vi "orderbook.test.Reduce.Size.1st.of.2.vi"(8 "error in":errorcluster) -> (0 "error out":errorcluster, 3 "Passed":bool)   [LabVIEW 2022 SP3]
uses:
  fpga/common/orderbook.command.type.ctl
  fpga/common/orderbook.command.ctl
  fpga/app/orderbook.result.type.ctl
  fpga/app/orderbook.entry.ctl
panel:
  out "Counters":T1
  out "OrderBook.Entries":T2[](array[typedef]) {"Side (U8)" format="%.0x"}
  in  "OrderBook.Command[]\nto Send":T4[](array[typedef])=[{"OrderBook Command.Type"=enum."AddOrder", "Side (U8)"=66, "Order Id (U64)"=336, "Quantity (U32)"=130, "Symbol (U64)"=29033, "Price (U64)"=9525, "Executed Quantity (U32)"=0, "Canceled Quantity (U32)"=0, "Remaining Quantity (U32)"=0, "Seconds (U64)"=0, "Nanoseconds (U64)"=0}, {"OrderBook Command.Type"=enum."AddOrder", "Side (U8)"=66, "Order Id (U64)"=337, "Quantity (U32)"=225, "Symbol (U64)"=29033, "Price (U64)"=9115, "Executed Quantity (U32)"=0, "Canceled Quantity (U32)"=0, "Remaining Quantity (U32)"=0, "Seconds (U64)"=0, "Nanoseconds (U64)"=0}, {"OrderBook Command.Type"=enum."ReduceSize", "Side (U8)"=66, "Order Id (U64)"=337, "Quantity (U32)"=0, "Symbol (U64)"=0, "Price (U64)"=0, "Executed Quantity (U32)"=0, "Canceled Quantity (U32)"=25, "Remaining Quantity (U32)"=0, "Seconds (U64)"=0, "Nanoseconds (U64)"=0}, {"OrderBook Command.Type"=enum."Get.All.Orders", "Side (U8)"=0, "Order Id (U64)"=0, "Quantity (U32)"=0, "Symbol (U64)"=0, "Price (U64)"=0, "Executed Quantity (U32)"=0, "Canceled Quantity (U32)"=0, "Remaining Quantity (U32)"=0, "Seconds (U64)"=0, "Nanoseconds (U64)"=0}] {"Side (U8)" format="%.0x"; "Order Id (U64)" format="%.0x"; "Symbol (U64)" format="%.0x"}
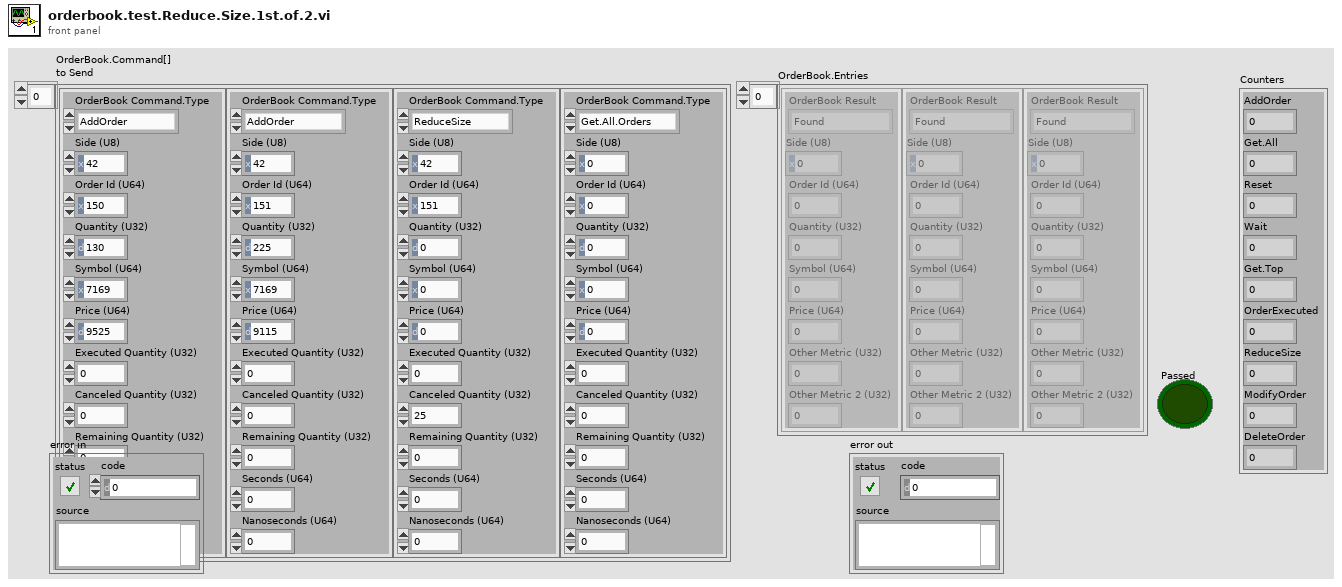
[diagram p1: front panel]
types:
  T1 = cluster{"AddOrder":u32, "Get.All":u32, "Reset":u32, "Wait":u32, "Get.Top":u32, "OrderExecuted":u32, "ReduceSize":u32, "ModifyOrder":u32, "DeleteOrder":u32}
  T2 = typedef "orderbook.entry.ctl" = cluster{"OrderBook Result":T3, "Side (U8)":u8, "Order Id (U64)":u64, "Quantity (U32)":u32, "Symbol (U64)":u64, "Price (U64)":u64, "Other Metric (U32)":u32, "Other Metric 2 (U32)":u32}
  T3 = typedef "orderbook.result.type.ctl" = enum16{"Found", "Not.Found"}
  T4 = typedef "orderbook.command.ctl" = cluster{"OrderBook Command.Type":T5, "Side (U8)":u8, "Order Id (U64)":u64, "Quantity (U32)":u32, "Symbol (U64)":u64, "Price (U64)":u64, "Executed Quantity (U32)":u32, "Canceled Quantity (U32)":u32, "Remaining Quantity (U32)":u32, "Seconds (U64)":u64, "Nanoseconds (U64)":u64}
  T5 = typedef "orderbook.command.type.ctl" = enum16{"Time", "AddOrder", "OrderExecuted", "OrderExecutedAtPrice", "ReduceSize", "ModifyOrder", "DeleteOrder", "Get.State", "Get.All.Orders", "Get.Top"}
  T6 = cluster{"Write.Request":bool, "Read.Request":bool, "Read.Address":u32, "Read.OrderBook.Entry":cluster{"OrderBook Result":enum16{"Found", "Not.Found"}, "Side (U8)":u8, "Order Id (U64)":u64, "Quantity (U32)":u32, "Symbol (U64)":u64, "Price (U64)":u64, "Other Metric (U32)":u32, "Other Metric 2 (U32)":u32}, "Number.of.Entries":u32, "OrderBook.State":enum16{"Reset", "Wait", "Get.Top", "Get.All.Orders", "AddOrder", "Order.Executed", "Reduce.Size", "Modify.Order", "Delete.Order"}, "Ready.For.OrderBook.Command":bool, "Memory.State":enum16{"New", "Request.Data", "Append", "Data.Ready"}, "Move":bool, "Read.Valid":bool, "Write.Address":u32, "Write.OrderBook.Entry":cluster{"OrderBook Result":enum16{"Found", "Not.Found"}, "Side (U8)":u8, "Order Id (U64)":u64, "Quantity (U32)":u32, "Symbol (U64)":u64, "Price (U64)":u64, "Other Metric (U32)":u32, "Other Metric 2 (U32)":u32}, "OrderBook.Result.Valid":bool, "Append":bool, "Counters":cluster{"AddOrder":u32, "Get.All":u32, "Reset":u32, "Wait":u32, "Get.Top":u32, "OrderExecuted":u32, "ReduceSize":u32, "ModifyOrder":u32, "DeleteOrder":u32}}
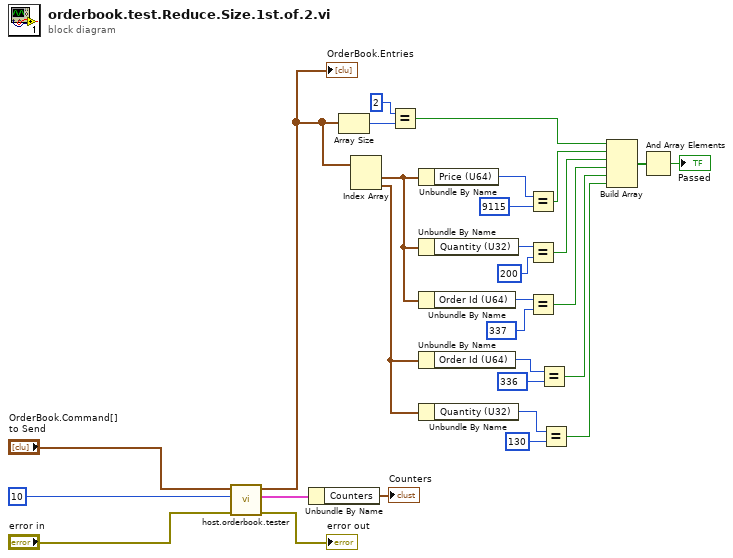
[diagram p0: block diagram]
diagram:
  n1 = call "host.orderbook.tester.vi"("error in"="error in", "Seconds to Wait"=10 ("Seconds\nto\nWait"), "OrderBook.Command[]\nto Send"="OrderBook.Command[]\nto Send") -> ("error out"=→"error out":errorcluster, "OrderBook.Variables"=w8:T6, "OrderBook.Entries"=w18:T2[])  [unwired: 6 in]
  "OrderBook.Entries" <- w18
  n2 = Unbundle By Name(w8) -> ("Counters"=→"Counters":T1)
  n3 = Array Size(array=w18) -> (size(s)=w26:i32)
  n4 = Index Array(array=w18) -> (element #1=w10:T2, element #2=w5:T2)  [unwired: 2 in]
  n5 = Equal?(x=2, y=w26) -> (x = y?=w21:bool)
  n6 = Unbundle By Name(w10) -> ("Price (U64)"=w23:u64)
  n7 = Unbundle By Name(w10) -> ("Quantity (U32)"=w16:u32)
  n8 = Unbundle By Name(w10) -> ("Order Id (U64)"=w14:u64)
  n9 = Unbundle By Name(w5) -> ("Order Id (U64)"=w7:u64)
  n10 = Unbundle By Name(w5) -> ("Quantity (U32)"=w4:u32)
  n11 = Equal?(x=w23, y=u64 9115) -> (x = y?=w22:bool)
  n12 = Equal?(x=w16, y=u32 200) -> (x = y?=w13:bool)
  n13 = Equal?(x=w14, y=u64 337) -> (x = y?=w12:bool)
  n14 = Equal?(x=w7, y=u64 336) -> (x = y?=w2:bool)
  n15 = Equal?(x=w4, y=u32 130) -> (x = y?=w1:bool)
  n16 = Build Array(w21, w22, w13, w12, w2, w1) -> (w20:bool[])
  n17 = And Array Elements(Boolean array=w20) -> (logical AND=→"Passed":bool)
